vi "Init_SubVI.vi"(8 "error in (no error)":errorcluster, 10 "Wave Analyzer":refnum<visa-resource-name>="Wave_Analyzer") -> (0 "error out":errorcluster)   [LabVIEW 2023]
uses:
  <instrlib>/Keysight XSAn/Keysight XSAn.lvlib
  KeysightN9020B.lvlib
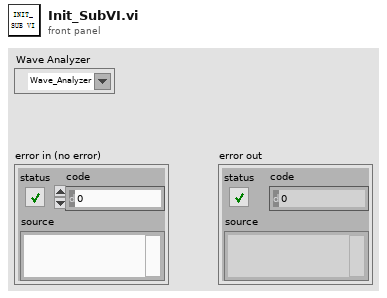
[diagram p1: front panel]
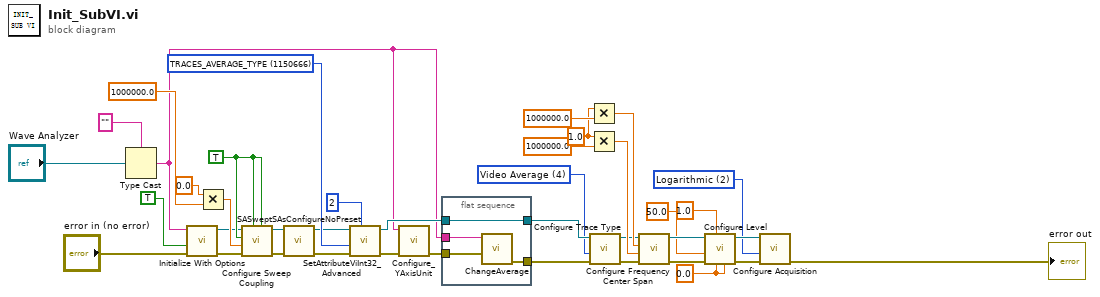
[diagram p0: block diagram]
diagram:
  w1 = 1.0 ("x")
  w5 = 0.0 ("reference level offset")
  w6 = 2 items=["Linear"=1, "Logarithmic"=2] ("vertical scale (Linear)")
  w22 = u32 1150666 items=["IVILXISYNC_ARM_ALARM_REPEAT_COUNT"=1950004, "IVILXISYNC_ARM_COUNT"=1950007, "IVILXISYNC_ARM_SOURCE_DETECTION"=1950010, "IVILXISYNC_EVENT_DRIVE_MODE"=1950030, "IVILXISYNC_EVENT_SLOPE"=1950031, "IVILXISYNC_EVENT_WIRED_OR_BIAS_MODE"=1950033, "IVILXISYNC_TRIGGER_ALARM_REPEAT_COUNT"=1950018, "IVILXISYNC_TRIGGER_COUNT"=1950021, "IVILXISYNC_TRIGGER_SOURCE_DETECTION"=1950025, "LEVEL_ATTENUATION_OPTIMIZE"=1150012, "LEVEL_ATTENUATION_STEP_INCREMENT"=1150013, "LEVEL_ELECTRONIC_ATTENUATION"=1150578, "MEMORYOPERATION_SCREEN_IMAGE_THEME"=1150678, "NUMBER_OF_SWEEPS"=1250010, "OUTPUT_ANALOG_TYPE"=1150679, "OUTPUT_AUXILIARY_IF_TYPE"=1150681, "PRESELECTOR_MW_PATH"=1150585, "RADIO_BAND_CLASS"=1150550, "RADIO_DEVICE"=1150547, "RADIO_NON_STANDARD_MEASUREMENT_ENABLED"=1150549, "RADIO_PACKET_TYPE"=1150551, "RADIO_STANDARD"=1150548, "REFOSCILLATOR_EXTERNAL_BANDWIDTH"=1150539, "REFOSCILLATOR_EXTERNAL_COUPLING"=1150538, "REFOSCILLATOR_SOURCE "=1150877, "STATETRIGGER_DETECTION"=1150159, "SYSTEM_IO_TIMEOUT"=1150783, "SYSTEM_TIMEOUT_MILLISECONDS"=1150175, "TRACE_DETECTOR_TYPE"=1150782, "TRACE_TYPE"=1250020, "TRACES_AVERAGE_TYPE"=1150666, "TRIGGER_EXTERNAL2_SLOPE"=1150671, "TRIGGER_EXTERNAL_SLOPE"=1150803, "TRIGGER_FRAME_SYNC_SOURCE"=1150841, "TRIGGER_LINE_DELAY_SLOPE"=1150836, "TRIGGER_RFBURST_SLOPE "=1150830, "TRIGGER_SOURCE"=1250301, "TRIGGER_VIDEO_SLOPE"=1150806, "VERTICAL_SCALE"=1250021, "VIDEO_TRIGGER_SLOPE"=1250502] ("AttributeID")
  w21 = 4 items=["Clear Write"=1, "Maximum Hold"=2, "Minimum Hold"=3, "Video Average"=4, "View"=5, "Store"=6] ("trace type (Clear Write)")
  w33 = TRUE ("resolution bandwidth auto (Off)")
  n1 = Type Cast(type="" ("resource string"), x="Wave Analyzer") -> (*(type *) &x=w18:string)
  n2 = call <instrlib>:"Initialize With Options.vi"("error in (no error)"="error in (no error)", "reset device (Off)"=TRUE, "resource string"=w18) -> ("error out"=w11:errorcluster, "instrument handle out"=w32:refnum<k15>)  [unwired: 7 in]
  n3 = Multiply(x=0.0, y=1000000.0) -> (x*y=w36:dbl)
  n4 = call <instrlib>:"Configure Sweep Coupling.vi"("sweep time auto (Off)"=w33, "video bandwidth auto (Off)"=w33, "error in (no error)"=w11, "resolution bandwidth"=w36, "resolution bandwidth auto (Off)"=w33, "instrument handle"=w32) -> ("error out"=w38:errorcluster, "instrument handle out"=w37:refnum<k15>)  [unwired: 4 in]
  n5 = call <instrlib>:"SASweptSAsConfigureNoPreset.vi"("error in (no error)"=w38, "instrument handle"=w37) -> ("error out"=w20:errorcluster, "instrument handle out"=w19:refnum<k15>)  [unwired: 8 in]
  n6 = call <instrlib>:"SetAttributeViInt32_Advanced.vi"("AttributeValue"=2, "error in (no error)"=w20, "AttributeID"=w22, "instrument handle"=w19) -> ("error out"=w26:errorcluster, "instrument handle out"=w24:refnum<k15>)  [unwired: 6 in]
  n7 = call "Configure_YAxisUnit.vi"("error in (no error)"=w26, "VISA resource name"=w18) -> ("error out"=w25:errorcluster)  [unwired: 9 in]
  n8 = flat-sequence {
    tunnel: w25 -> [w43]
    tunnel: [w42] -> w28
    tunnel: w24 -> [w41]
    tunnel: [w41] -> w27
    tunnel: w18 -> [w40]
    frame #0 {
      n9 = call "ChangeAverage.vi"("error in (no error)"=w43, "VISA resource name"=w40) -> ("error out"=w42:errorcluster)  [unwired: 9 in]
    }
  }
  n10 = Multiply(x=w1, y=1000000.0) -> (x*y=w17:dbl)
  n11 = Multiply(x=w1, y=1000000.0) -> (x*y=w16:dbl)
  n12 = call <instrlib>:"Configure Trace Type.vi"("error in (no error)"=w28, "trace type (Clear Write)"=w21, "instrument handle"=w27) -> ("error out"=w13:errorcluster, "instrument handle out"=w12:refnum<k15>)  [unwired: 7 in]
  n13 = call <instrlib>:"Configure Frequency Center Span.vi"("error in (no error)"=w13, "span"=w16, "center frequency"=w17, "instrument handle"=w12) -> ("error out"=w7:errorcluster, "instrument handle out"=w8:refnum<k15>)  [unwired: 6 in]
  n14 = call <instrlib>:"Configure Level.vi"("attenuation"=w5, "reference level offset"=w5, "reference level"=1.0 ("reference level offset"), "error in (no error)"=w7, "input impedance"=50.0, "instrument handle"=w8) -> ("error out"=w9:errorcluster, "instrument handle out"=w10:refnum<k15>)  [unwired: 4 in]
  n15 = call <instrlib>:"Configure Acquisition.vi"("error in (no error)"=w9, "vertical scale (Linear)"=w6, "instrument handle"=w10) -> ("error out"=→"error out":errorcluster)  [unwired: 7 in, 1 out]
